vi "UHR-Fleezers Control (host) - 12.0.vi"() -> ()   [LabVIEW 2012] (continued)
      event "Reset Trap Pos. FB": Value Change {
        n2500 = event-data() -> ()  [unwired: 7 out]
        n2501 = xnode "Read/Write Control"("FPGA VI Reference In"=w4144, "error in"=w4143, "Trap Pos. FB Reset"="Reset Trap Pos. FB") -> ()  [unwired: 2 out]
      }
      event "Rem fb disp offset": Value Change {
        n2502 = event-data() -> ()  [unwired: 7 out]
        n2503 = local write "Rem fb disp offset"(FALSE ("Rem fb disp offset")) -> ()
        n2504 = local read "Mean T1 Position (nm)"() -> (w4146:dbl)
        n2505 = local read "FB Trap Pos Offset"() -> (w4147:dbl)
        n2506 = Subtract(x=w4147, y=w4146) -> (x-y=w4145:dbl)
        n2507 = local write "FB Trap Pos Offset"(w4145) -> ()
      }
      event "Threshold (nm)": Value Change {
        n2508 = event-data() -> ()  [unwired: 7 out]
        n2509 = flat-sequence {
          tunnel: w4151 -> [w4159]
          tunnel: w4150 -> [w4158]
          tunnel: [w4152] -> w4149
          tunnel: w4149 -> [w4165]
          frame #0 {
            n2510 = xnode "Read/Write Control"("FPGA VI Reference In"=w4159, "error in"=w4158) -> ("FPGA VI Reference Out"=w4155:T19, "error out"=w4154:errorcluster, "FPGA TTrig Thresh"=w4156:i64)
            n2511 = local read "Threshold stored (nm)"() -> (w4164:dbl)
            n2512 = local read "Threshold (nm)"() -> (w4152:dbl)
            n2513 = local read "AOM X Cal (nm/MHz)"() -> (w4162:dbl)
            n2514 = Subtract(x=w4152, y=w4164) -> (x-y=w4163:dbl)
            n2515 = Divide(x=w4163, y=w4162) -> (x/y=w4160:dbl)
            n2516 = call "IR AOM freq to word.vi"("Frequency In (MHz)"=w4160) -> ("Frequency Word Out (double)"=w4161:dbl)
            n2517 = To Quad Integer(1:w4161) -> (0:w4157:i64)
            n2518 = Add(x=w4156, y=w4157) -> (x+y=w4153:i64)
            n2519 = xnode "Read/Write Control"("FPGA VI Reference In"=w4155, "error in"=w4154, "FPGA TTrig Thresh"=w4153) -> ()  [unwired: 2 out]
          }
          frame #1 {
            "Threshold stored (nm)" <- w4165
          }
        }
      }
      event "FB Trig Integrate": Value Change {
        n2520 = event-data() -> ()  [unwired: 7 out]
        n2521 = local read "FB Trig Integrate"() -> (w4167:u32)
        n2522 = xnode "Read/Write Control"("FPGA VI Reference In"=w4169, "error in"=w4168, "FB Trig Integrate"=w4167) -> ("error out"=w4166:errorcluster)  [unwired: 1 out]
      }
      event "11": Value Change {
        n2523 = event-data() -> ()  [unwired: 7 out]
        n2524 = local read "11"() -> (w4170:bool)
        n2525 = case shown="True" w4170 {
          frame False {
          }
          frame True {
            n2526 = local read "Messages"() -> (w4172:string)
            n2527 = call "Update messages.vi"("Message to add"="You kicked it up to 11!", "Old message string"=w4172) -> ("New message string"=w4173:string)
            n2528 = call <vilib>:"Beep.vi"() -> ()  [unwired: 12 in]
            n2529 = local write "Messages"(w4173) -> ()
          }
        }
      }
      event "Trap Pos. FB ON": Value Change {
        n2530 = event-data() -> ()  [unwired: 7 out]
        n2531 = xnode "Read/Write Control"("FPGA VI Reference In"=w4176, "error in"=w4175, "Force feedback"="Trap Pos. FB ON") -> ()  [unwired: 2 out]
      }
      event "Remove Action Offset": Value Change {
        n2532 = event-data() -> ()  [unwired: 7 out]
        n2533 = local write "Remove Action Offset"(FALSE ("Remove Action Offset")) -> ()
        n2534 = local read "Trap Pos. FB Mult Factor"() -> (w4181:i64)
        n2535 = local read "Trap Pos FB Action"() -> (w4179:i64)
        n2536 = local read "Trap Pos. FB Offset Factor"() -> (w4177:i64)
        n2537 = Multiply(x=w4181, y=w4179) -> (x*y=w4180:i64)
        n2538 = Add(x=w4180, y=w4177) -> (x+y=w4178:i64)
        n2539 = local write "Trap Pos. FB Offset Factor"(w4178) -> ()
        n2540 = xnode "Read/Write Control"("FPGA VI Reference In"=w4184, "error in"=w4183, "Trap Pos. FB Offset Factor"=w4178) -> ()  [unwired: 2 out]
      }
      event "Remove Unwinding Offset": Value Change {
        n2541 = event-data() -> ()  [unwired: 7 out]
        n2542 = local write "Remove Unwinding Offset"(FALSE ("Remove Action Offset")) -> ()
        n2543 = local read "Trap Pos. FB Mult Factor"() -> (w4196:i64)
        n2544 = local read "Trap Pos FB Action"() -> (w4194:i64)
        n2545 = local read "Trap Pos. FB Offset Factor"() -> (w4193:i64)
        n2546 = Multiply(x=w4196, y=w4194) -> (x*y=w4195:i64)
        n2547 = local read "Trap Pos. FB Mult Factor"() -> (w4192:i64)
        n2548 = Add(x=w4195, y=w4193) -> (x+y=w4186:i64)
        n2549 = Multiply(x=32768, y="factor") -> (x*y=w4189:dbl)
        n2550 = Multiply(x=w4189, y=w4192) -> (x*y=w4191:dbl)
        n2551 = Subtract(x=w4186, y=w4191) -> (x-y=w4190:dbl)
        n2552 = To Quad Integer(1:w4190) -> (0:w4185:i64)
        n2553 = xnode "Read/Write Control"("FPGA VI Reference In"=w4199, "error in"=w4198, "Trap Pos. FB Offset Factor"=w4185) -> ()  [unwired: 2 out]
        n2554 = local write "Trap Pos. FB Offset Factor"(w4185) -> ()
      }
      event "Trap Pos. FB Range", "Trap Pos. FB Gains", "Trap Pos. FB Mult Factor", "Trap Pos. FB Offset Factor", "Trap Pos FB Negate Action", "Trap Pos FB Monitor\nT1 or T2", "Differential FB?", "Negate Diff?": Value Change {
        n2555 = event-data() -> ()  [unwired: 7 out]
        n2556 = local read "Negate Diff?"() -> (w4200:bool)
        n2557 = xnode "Read/Write Control"("FPGA VI Reference In"=w4210, "error in"=w4209, "Trap Pos. FB Range"="Trap Pos. FB Range", "Trap Pos. FB Gains"="Trap Pos. FB Gains", "Trap Pos. FB Mult Factor"="Trap Pos. FB Mult Factor", "Trap Pos. FB Offset Factor"="Trap Pos. FB Offset Factor", "Trap Pos FB Negate Action"="Trap Pos FB Negate Action", "Trap Pos FB Monitor T1 or T2"="Trap Pos FB Monitor\nT1 or T2", "AI1 X Scale"="Trap Pos. AI1 X Pre-scale", "Negate Diff?"=w4200, "Diff FB Measurement?"="Differential FB?") -> ()  [unwired: 2 out]
      }
      event "Trap Pos FB SP", "Trap Pos FB SP 2", "Use SP 2": Value Change {
        n2558 = event-data() -> ()  [unwired: 7 out]
        n2559 = Select(t="Trap Pos FB SP 2", s="Use SP 2", f="Trap Pos FB SP") -> (s? t:f=w4211:fxp<+/-,16,1>)
        n2560 = xnode "Read/Write Control"("FPGA VI Reference In"=w4216, "error in"=w4215, "Trap Pos. FB SP"=w4211) -> ()  [unwired: 2 out]
      }
      event "Offset SP2 from SP1": Value Change {
        n2561 = event-data() -> ()  [unwired: 7 out]
        n2562 = local read "Trap Pos FB SP"() -> (w4219:fxp<+/-,16,1>)
        n2563 = Add(x=w4219, y="SP2 Offset") -> (x+y=w4217:fxp<+/-,16,1>)
        n2564 = property on="Trap Pos FB SP 2" class="DigNum (strict)"("Val(Sgnl)"=w4217) -> ()  [unwired: 2 in, 2 out]
        n2565 = local write "Offset SP2 from SP1"(FALSE ("Offset SP2 from SP1")) -> ()
      }
      event "Set Reading to\nSetpoint": Value Change {
        # "This is the actual PID input signal"
        n2566 = event-data() -> ()  [unwired: 7 out]
        n2567 = local write "Set Reading to\nSetpoint"(FALSE ("Set SP to Reading")) -> ()
        n2568 = xnode "Read/Write Control"("FPGA VI Reference In"=w4225, "error in"=w4224) -> ("FPGA VI Reference Out"=w4223:T19, "error out"=w4222:errorcluster, "Trap Pos FB Int-Norm Signal"=w4221:fxp<+/-,16,1>)
        n2569 = local read "Differential FB?"() -> (w4226:bool)
        n2570 = case shown="False" w4226 {
          tunnel: [w4231 w4238] -> w4228
          tunnel: w4221 -> [w4229 w4238]
          frame False {
            n2571 = local read "Trap Pos FB Monitor\nT1 or T2"() -> (w4234:bool)
            n2572 = local read "Trap X AI1 (DMA)"() -> (w4237:T13)
            n2573 = Unbundle By Name(w4237) -> ("Set 1"=w4236:fxp<+/-,16,1>, "Set 2"=w4235:fxp<+/-,16,1>)
            n2574 = Select(t=w4236, s=w4234, f=w4235) -> (s? t:f=w4233:fxp<+/-,16,1>)
            n2575 = Not(x="Set SP Using...") -> (.not. x?=w4230:bool)
            n2576 = Select(t=w4229, s=w4230, f=w4233) -> (s? t:f=w4231:fxp<+/-,16,1>)
          }
          frame True {
          }
        }
        n2577 = xnode "Read/Write Control"("FPGA VI Reference In"=w4223, "error in"=w4222, "Trap Pos. FB SP"=w4228) -> ()  [unwired: 2 out]
        n2578 = local write "Trap Pos FB SP"(w4228) -> ()
      }
      event "Trap Pos. FB Out Scale 2^n": Value Change {
        n2579 = event-data() -> ()  [unwired: 7 out]
        n2580 = Scale By Power Of 2(n="Trap Pos. FB Out Scale 2^n", x=ext 1.0) -> (x*2^n=w4239:ext)
        n2581 = property on="Trap Pos. FB Mult Factor" class="DigNum (strict)"("Val(Sgnl)"=w4239) -> ()  [unwired: 2 in, 2 out]
      }
      event "Trap Pos FB Int Count": Value Change {
        n2582 = event-data() -> ()  [unwired: 7 out]
        n2583 = xnode "Read/Write Control"("FPGA VI Reference In"=w4244, "error in"=w4243, "Trap Pos FB Int Count"="Trap Pos FB Int Count") -> ()  [unwired: 2 out]
      }
      event "Trap pos": Value Change {
        n2584 = event-data() -> ()  [unwired: 7 out]
        n2585 = case shown="True" "Trap pos" {
          frame False {
            n2586 = property on="Trap Delta Graph" class="WFGraph (strict)"("Visible"=TRUE) -> ()  [unwired: 2 in, 2 out]
            n2587 = property on="Saved trap pos" class="WFGraph (strict)"("Visible"=FALSE) -> ()  [unwired: 2 in, 2 out]
          }
          frame True {
            n2588 = property on="Saved trap pos" class="WFGraph (strict)"("Visible"=TRUE) -> ()  [unwired: 2 in, 2 out]
            n2589 = property on="Trap Delta Graph" class="WFGraph (strict)"("Visible"=FALSE) -> ()  [unwired: 2 in, 2 out]
          }
        }
      }
    }
    "error out 2" <- w3149
    n2590 = node-c288() -> ()  [unwired: 2 out]
  }
  n2591 = timed-loop "Oscillate Trap/AOM (fishing, debugging)" {
    tunnel: w6 -> [w4251]
    tunnel: [w4250] -> w100
    timing: w95 -> [_]
    timing-out: [_] -> w94
    stop <- w4250 stop-if-true
    n2592 = node-c288() -> ()  [unwired: 2 out]
    n2593 = event shown="[0] \"Oscillate Set 1\", \"Fish for Tether\": Value Change" {
      selector: _ -> [_ _ _]
      dyn-events: _ -> [_ _ _]
      timeout: _ -> [_ _ _]
      tunnel: w4251 -> [w4258 _ _]
      tunnel: [FALSE ("Stop All") _ w4847] -> w4250
      event "Oscillate Set 1", "Fish for Tether": Value Change {
        n2594 = event-data() -> ()  [unwired: 6 out]
        n2595 = local read "Oscillate Set 1"() -> (w4257:bool)
        n2596 = Or(x=w4257, y="Fish for Tether") -> (x .or. y?=w4255:bool)
        n2597 = case shown="True" w4255 {
          tunnel: w4258 -> [_ w4261]
          tunnel: "Fish for Tether" -> [_ w4260]
          frame False {
          }
          frame True {
            n2598 = case shown="True" w4260 {
              selector: w4260 -> [w4264 w4270]
              tunnel: [w4264 w4270] -> w4259
              frame False {
              }
              frame True {
                n2599 = local write "Scan axis 2"(TRUE) -> ()
                n2600 = local write "Tether"(FALSE ("Tether")) -> ()
                n2601 = local read "Flow ON during cal?"() -> (w4265:bool)
                n2602 = property on="Trap Delta (MHz)" class="DigNum (strict)"("Val(Sgnl)"="Furthest Delta (MHz)") -> ()  [unwired: 2 in, 2 out]
                n2603 = Or(x="Flow ON during \nfishing?", y=w4265) -> (x .or. y?=w4266:bool)
                n2604 = Wait (ms)(milliseconds to wait=u32 500) -> ()  [unwired: 1 out]
                n2605 = property on="Sample Channel\nFlow" class="Bool (strict)"("Val(Sgnl)"=w4266) -> ()  [unwired: 2 in, 2 out]
              }
            }
            n2606 = node-c288() -> (w4263:T21)  [unwired: 4 out]
            n2607 = timed-loop "Oscillate AOD" {
              timing: w4263 -> [_]
              timing-out: [_] -> w4262
              tunnel: w4261 -> [w4280]
              tunnel: w4259 -> [w4273]
              i -> [w4282]
              stop <- w4279 stop-if-true
              n2608 = node-c288() -> (w4281:i64)  [unwired: 1 out]
              n2609 = flat-sequence {
                tunnel: w4282 -> [w4309]
                tunnel: w4281 -> [w4308]
                tunnel: w4280 -> [w4287]
                tunnel: w4273 -> [w4290]
                tunnel: [w4290] -> w4278
                tunnel: [w4289] -> w4277
                tunnel: [w4286] -> w4276
                tunnel: [w4283] -> w4274
                tunnel: w4278 -> [w4345]
                tunnel: w4277 -> [w4343]
                tunnel: w4276 -> [w4342]
                tunnel: [w4341] -> w4275
                tunnel: w4274 -> [w4340]
                tunnel: [w4417] -> w4279
                tunnel: w4275 -> [w4416]
                frame #0 {
                  n2610 = Divide(x=w4308, y=i64 1000) -> (x/y=w4303:dbl)
                  n2611 = Multiply(x=w4303, y=w4309) -> (x*y=w4305:dbl)
                  n2612 = local read "BD 1 Frequency 2 (MHz)"() -> (w4288:dbl)
                  n2613 = Multiply(x="Osc. freq. (Hz)", y=6.283185307179586) -> (x*y=w4306:dbl)
                  n2614 = Multiply(x=w4306, y=w4305) -> (x*y=w4285:dbl)
                  n2615 = local read "BD 1 Frequency 1 (MHz)"() -> (w4293:dbl)
                  n2616 = local read "BD 2 Frequency 1 (MHz)"() -> (w4292:dbl)
                  n2617 = case shown="True" w4290 {
                    tunnel: w4285 -> [w4315 w4320]
                    tunnel: w4293 -> [_ w4331]
                    tunnel: w4288 -> [_ w4332]
                    tunnel: [w4312 w4326] -> w4291
                    tunnel: [FALSE w4323] -> w4286
                    tunnel: [0.0 w4316] -> w4283
                    frame False {
                      n2618 = Sine(x=w4315) -> (sin(x)=w4313:dbl)
                      n2619 = Multiply(x=w4313, y="Osc. amp. (MHz)") -> (x*y=w4312:dbl)
                    }
                    frame True {
                      n2620 = Cosine(x=w4320) -> (cos(x)=w4335:dbl)
                      n2621 = Subtract(x=w4332, y=w4331) -> (x-y=w4330:dbl)
                      n2622 = Decrement(x=w4335) -> (x-1=w4334:dbl)
                      n2623 = Subtract(x=w4330, y="Closest Delta (MHz)") -> (x-y=w4327:dbl)
                      n2624 = Divide(x=w4334, y=-2.0) -> (x/y=w4328:dbl)
                      n2625 = Multiply(x=w4328, y=w4327) -> (x*y=w4326:dbl)
                      n2626 = local read "Vec Mean of T1 T2"() -> (w4322:dbl[])
                      n2627 = Greater?(x=w4322, y="Stop F (pN)") -> (0:w4324:bool[])
                      n2628 = Or Array Elements(Boolean array=w4324) -> (logical OR=w4323:bool)
                      n2629 = Divide(x=w4320, y=6.283185307179586) -> (x/y=w4319:dbl)
                      n2630 = Round Toward +Infinity(x=w4319) -> (ceil(x): smallest int >= x=w4316:dbl)
                      "Attempts" <- w4316
                      n2631 = Greater?(x=w4316, y="Attempt Limit") -> (0:w4318:bool)
                      n2632 = case shown="True" w4318 {
                        frame False {
                        }
                        frame True {
                          n2633 = local write "Fish for Tether"(FALSE ("Fish for Tether")) -> ()
                          n2634 = call <vilib>:"Beep.vi"() -> ()  [unwired: 3 in, 9 out]
                          n2635 = local read "Messages"() -> (w4337:string)
                          n2636 = call "Update messages.vi"("Message to add"="Tether fishing timeout." ("Messages"), "Old message string"=w4337) -> ("New message string"=→"Messages":string)
                        }
                      }
                    }
                  }
                  n2637 = Select(t=w4293, s="Scan axis 2", f=w4292) -> (s? t:f=w4296:dbl)
                  n2638 = Add(x=w4291, y=w4296) -> (x+y=w4289:dbl)
                  n2639 = Select(t=w4289, s="Scan axis 2", f=w4293) -> (s? t:f=w4299:dbl)
                  n2640 = Select(t=w4292, s="Scan axis 2", f=w4289) -> (s? t:f=w4298:dbl)
                  n2641 = local read "Y RF Frequency Limits (MHz)"() -> (w4294:T16)
                  n2642 = local read "X RF Frequency Limits (MHz)"() -> (w4295:T16)
                  n2643 = local read "BD 1 Frequency 3 (MHz)"() -> (w4302:dbl)
                  n2644 = local read "BD 2 Frequency 2 (MHz)"() -> (w4301:dbl)
                  n2645 = local read "BD 2 Frequency 3 (MHz)"() -> (w4300:dbl)
                  n2646 = call "set RF board frequency - interlace.vi"("Board 2 Frequency Limits"=w4294, "Board 1 Frequency Limits"=w4295, "FPGA VI Reference In"=w4287, "Board 2 Frequency 3 (MHz)"=w4300, "Board 1 Frequency 3 (MHz)"=w4302, "Board 2 Frequency 2 (MHz)"=w4301, "Board 2 Frequency 1 (MHz)"=w4298, "Board 1 Frequency 2 (MHz)"=w4288, "Board 1 Frequency 1  (MHz)"=w4299) -> ()  [unwired: 1 in, 2 out]
                }
                frame #1 {
                  n2647 = And(x=w4345, y=w4342) -> (x .and. y?=w4344:bool)
                  n2648 = case "Only if were fishing and now formed tether" shown="False" w4344 {
                    tunnel: w4343 -> [w4347 w4362]
                    tunnel: [w4346 w4361] -> w4341
                    tunnel: w4340 -> [_ w4357]
                    frame False {
                      n2649 = local read "Fish for Tether"() -> (w4346:bool)
                      n2650 = case shown="False" w4346 {
                        tunnel: w4347 -> [w4348 _]
                        frame False {
                          n2651 = property on="BD 1 Frequency 1 (MHz)" class="DigNum (strict)"("Val(Sgnl)"=w4348) -> ()  [unwired: 2 in, 2 out]
                        }
                        frame True {
                        }
                      }
                    }
                    frame True {
                      w4361 = FALSE ("Fish for Tether")
                      n2652 = call <vilib>:"Beep.vi"() -> ()  [unwired: 3 in, 9 out]
                      n2653 = Number To Decimal String(number=w4357, width (-)=i16 1) -> (decimal integer string=w4355:string)
                      n2654 = Concatenate Strings("Formed tether in ", w4355, " attempt(s)." ("string")) -> (w4352:string)
                      n2655 = local read "Messages"() -> (w4359:string)
                      n2656 = local write "Fish for Tether"(w4361) -> ()
                      n2657 = call "Update messages.vi"("Message to add"=w4352, "Old message string"=w4359) -> ("New message string"=w4358:string)
                      n2658 = local write "Messages"(w4358) -> ()
                      n2659 = Get Date/Time In Seconds() -> (seconds since 1Jan1904=→"Time tether formed":timestamp)
                      n2660 = local read "Flow ON during cal?"() -> (w4349:bool)
                      n2661 = property on="Sample Channel\nFlow" class="Bool (strict)"("Val(Sgnl)"=w4349) -> (error out=w4350:errorcluster)  [unwired: 2 in, 1 out]
                      n2662 = case shown="\"2\", \"3\", \"4\", \"5\", \"6\"" "Then..." {
                        selector: "Then..." -> [_ w4365]
                        tunnel: w4362 -> [w4364 _]
                        tunnel: w4350 -> [_ _]
                        frame "1", Default {
                          n2663 = property on="BD 1 Frequency 1 (MHz)" class="DigNum (strict)"("Val(Sgnl)"=w4364) -> ()  [unwired: 2 in, 2 out]
                        }
                        frame "2", "3", "4", "5", "6" {
                          n2664 = flat-sequence {
                            tunnel: w4365 -> [w4367]
                            frame #0 {
                              n2665 = property on="Trap Delta (MHz)" class="DigNum (strict)"("Val(Sgnl)"="Move to Delta 1 (MHz)") -> ()  [unwired: 2 in, 2 out]
                            }
                            frame #1 {
                              n2666 = case shown="\"5\", \"6\"" w4367 {
                                selector: w4367 -> [w4370 w4380 _]
                                frame "3", "4" {
                                n2667 = flat-sequence {
                                tunnel: w4370 -> [w4371]
                                tunnel: [w4371] -> w4368
                                tunnel: [w4373] -> w4369
                                tunnel: w4368 -> [w4373]
                                tunnel: w4369 -> [w4377]
                                frame #0 {
                                n2668 = property on="Green Laser ON/Interlacing" class="Bool (strict)"("Val(Sgnl)"=TRUE ("Value (Signaling)")) -> ()  [unwired: 2 in, 2 out]
                                }
                                frame #1 {
                                n2669 = Multiply(x="Wait Before Save (s)", y=u32 1000 ("x")) -> (x*y=w4375:u32)
                                n2670 = Wait (ms)(milliseconds to wait=w4375) -> ()  [unwired: 1 out]
                                }
                                frame #2 {
                                n2671 = property on="Start Saving" class="Bool (strict)"("Value"=TRUE ("Start Saving")) -> ()  [unwired: 2 in, 2 out]
                                n2672 = case shown="\"4\"" w4377 {
                                frame Default {
                                }
                                frame "4" {
                                n2673 = property on="Fl. Triggered..." class="Bool (strict)"("Val(Sgnl)"=TRUE ("Value (Signaling)")) -> ()  [unwired: 2 in, 2 out]
                                }
                                }
                                }
                                }
                                }
                                frame "5", "6" {
                                n2674 = stacked-sequence {
                                tunnel: w4380 -> [_ _ _ _ _ _ w4392]
                                frame #0 {
                                n2675 = Replace Array Subset(array=u32[] [0] ("Index Values"), new element="Raster Set Upon Tether", index=0) -> (w4381:u32[])
                                n2676 = property on="Saved AOD Raster Scan Parameter Sets" class="Arr (strict)"("Index Values"=w4381) -> ()  [unwired: 2 in, 2 out]
                                }
                                frame #1 {
                                n2677 = Wait (ms)(milliseconds to wait=u32 500) -> ()  [unwired: 1 out]
                                }
                                frame #2 {
                                n2678 = property on="Load parameters" class="Bool (strict)"("Val(Sgnl)"=TRUE ("Value (Signaling)")) -> ()  [unwired: 2 in, 2 out]
                                n2679 = case shown="True" "Green ON During Raster" {
                                frame False {
                                }
                                frame True {
                                n2680 = property on="Green Laser ON/Interlacing" class="Bool (strict)"("Val(Sgnl)"=TRUE ("Value (Signaling)")) -> ()  [unwired: 2 in, 2 out]
                                }
                                }
                                }
                                frame #3 {
                                n2681 = Wait (ms)(milliseconds to wait=u32 500) -> ()  [unwired: 1 out]
                                }
                                frame #4 {
                                n2682 = property on="Trap Raster Scan" class="Bool (strict)"("Val(Sgnl)"=TRUE ("Value (Signaling)")) -> ()  [unwired: 2 in, 2 out]
                                }
                                frame #5 {
                                n2683 = Wait (ms)(milliseconds to wait=u32 2000) -> ()  [unwired: 1 out]
                                }
                                frame #6 {
                                n2684 = flat-sequence {
                                tunnel: w4392 -> [w4399]
                                frame #0 {
                                n2685 = while {
                                stop <- w4395 stop-if-true
                                n2686 = local read "Raster Scanning..."() -> (w4394:bool)
                                n2687 = local read "Saving..."() -> (w4397:bool)
                                n2688 = Wait (ms)(milliseconds to wait=u32 100) -> ()  [unwired: 1 out]
                                n2689 = Not(x=w4397) -> (.not. x?=w4396:bool)
                                n2690 = Not(x=w4394) -> (.not. x?=w4393:bool)
                                n2691 = And(x=w4396, y=w4393) -> (x .and. y?=w4395:bool)
                                }
                                }
                                frame #1 {
                                n2692 = local read "Tether"() -> (w4400:bool)
                                n2693 = case shown="True" w4400 {
                                tunnel: w4399 -> [_ w4402]
                                frame False {
                                n2694 = property on="Fish for Tether" class="Bool (strict)"("Val(Sgnl)"="Fish again after \nraster break?") -> ()  [unwired: 2 in, 2 out]
                                }
                                frame True {
                                n2695 = stacked-sequence {
                                tunnel: w4402 -> [_ w4406 _ _]
                                frame #0 {
                                n2696 = property on="Trap Delta (MHz)" class="DigNum (strict)"("Val(Sgnl)"="Move to Delta 2 (MHz)") -> ()  [unwired: 2 in, 2 out]
                                n2697 = case shown="True" "Flow ON after\ntether testing?" {
                                frame False {
                                }
                                frame True {
                                n2698 = property on="Sample Channel\nFlow" class="Bool (strict)"("Val(Sgnl)"=TRUE ("Value (Signaling)")) -> ()  [unwired: 2 in, 2 out]
                                }
                                }
                                }
                                frame #1 {
                                n2699 = flat-sequence {
                                tunnel: w4406 -> [w4408]
                                frame #0 {
                                n2700 = Wait (ms)(milliseconds to wait=u32 500) -> ()  [unwired: 1 out]
                                }
                                frame #1 {
                                n2701 = case shown="\"6\"" w4408 {
                                frame Default {
                                }
                                frame "6" {
                                n2702 = property on="Green Laser ON/Interlacing" class="Bool (strict)"("Val(Sgnl)"=TRUE ("Green Laser ON/Interlacing")) -> ()  [unwired: 2 in, 2 out]
                                }
                                }
                                }
                                frame #2 {
                                n2703 = Wait (ms)(milliseconds to wait=u32 500) -> ()  [unwired: 1 out]
                                }
                                frame #3 {
                                n2704 = local write "Start Saving"("Save at end (5, 6)") -> ()
                                }
                                }
                                }
                                frame #2 {
                                n2705 = local read "Bead Sep. Int. Time (s)"() -> (w4414:dbl)
                                n2706 = Multiply(x=w4414, y=1000.0) -> (x*y=w4413:dbl)
                                n2707 = Wait (ms)(milliseconds to wait=w4413) -> ()  [unwired: 1 out]
                                }
                                frame #3 {
                                n2708 = property on="Remove Offset" class="Bool (strict)"("Val(Sgnl)"=TRUE ("Value (Signaling)")) -> ()  [unwired: 2 in, 2 out]
                                }
                                }
                                }
                                }
                                }
                                }
                                }
                                }
                                }
                                frame "2", Default {
                                }
                              }
                            }
                          }
                        }
                      }
                      "Tether" <- "Tether Alarm?"
                    }
                  }
                }
                frame #2 {
                  n2709 = local read "Oscillate Set 1"() -> (w4421:bool)
                  n2710 = local read "Stop All"() -> (w4419:bool)
                  n2711 = Or(x=w4421, y=w4416) -> (x .or. y?=w4418:bool)
                  n2712 = Not(x=w4418) -> (.not. x?=w4420:bool)
                  n2713 = Compound Arithmetic op=OR(w4419, w4420) -> (w4417:bool)
                }
              }
              n2714 = node-c288() -> ()  [unwired: 2 out]
            }
            n2715 = node-c288(w4262) -> ()  [unwired: 1 out]
          }
        }
      }
      event "Fl. Triggered...": Value Change {
        n2716 = event-data() -> ()  [unwired: 7 out]
        n2717 = case shown="True" "Fl. Triggered..." {
          frame False {
          }
          frame True {
            n2718 = node-c288() -> (w4432:T21)  [unwired: 4 out]
            n2719 = timed-loop {
              timing: w4432 -> [_]
              timing-out: [_] -> w4431
              tunnel: "Action" -> [w4440]
              shift-right: [w4437] -> _
              shift-left: u8 255 -> [w4439]
              shift-right: [w4434] -> _
              shift-left: 255 -> [w4436]
              stop <- w4433 stop-if-true
              # "Reset confocal spot"
              n2720 = node-c288() -> ()  [unwired: 2 out]
              n2721 = flat-sequence {
                tunnel: w4440 -> [w4460]
                tunnel: w4439 -> [w4459]
                tunnel: [w4458] -> w4438
                tunnel: w4436 -> [w4445]
                tunnel: [w4444] -> w4435
                tunnel: [w4839] -> w4433
                tunnel: w4438 -> [w4838]
                tunnel: [w4838] -> w4437
                tunnel: [w4837] -> w4434
                tunnel: w4435 -> [w4837]
                frame #0 {
                  n2722 = local read "Delta Fl. 2"() -> (w4457:dbl)
                  n2723 = local read "Delta Fl. 1"() -> (w4452:dbl)
                  n2724 = Multiply(x="Fl. Delta Thresh. (kHz)", y=1000.0) -> (x*y=w4447:dbl)
                  n2725 = Select(t=w4452, s="APD to Watch", f=w4457) -> (s? t:f=w4448:dbl)
                  n2726 = Greater?(x=w4448, y=w4447) -> (0:w4453:bool)
                  n2727 = Or(x="Force Yank", y=w4453) -> (x .or. y?=w4451:bool)
                  n2728 = And(x=w4451, y="Yank when?") -> (x .and. y?=w4449:bool)
                  n2729 = case shown="False" w4449 {
                    tunnel: w4460 -> [w4463 w4664]
                    tunnel: w4459 -> [w4465 w4660]
                    tunnel: [w4465 w4658] -> w4458
                    tunnel: w4448 -> [w4471 _]
                    tunnel: w4447 -> [w4470 _]
                    tunnel: "Force Yank" -> [w4468 _]
                    tunnel: w4445 -> [w4467 w4657]
                    tunnel: [w4466 w4657] -> w4444
                    frame False {
                      n2730 = Negate(x=w4470) -> (-x=w4462:dbl)
                      n2731 = local write "Fl. High"(TRUE ("Fl. High")) -> ()
                      n2732 = Less?(x=w4471, y=w4462) -> (x < y?=w4469:bool)
                      n2733 = Or(x=w4468, y=w4469) -> (x .or. y?=w4464:bool)
                      n2734 = case shown="True" w4464 {
                        tunnel: w4467 -> [w4472 w4482]
                        tunnel: [w4472 w4481] -> w4466
                        tunnel: w4463 -> [_ w4480]
                        frame False {
                        }
                        frame True {
                          n2735 = flat-sequence {
                            tunnel: w4482 -> [w4488]
                            tunnel: w4480 -> [w4485]
                            tunnel: [w4487] -> w4479
                            tunnel: [w4486] -> w4478
                            tunnel: [w4485] -> w4477
                            tunnel: w4476 -> [w4484]
                            tunnel: [w4484] -> w4475
                            tunnel: w4474 -> [w4483]
                            tunnel: [w4483] -> w4473
                            tunnel: [w4559] -> w4481
                            tunnel: w4479 -> [w4559]
                            tunnel: w4478 -> [w4558]
                            tunnel: w4477 -> [w4557]
                            tunnel: w4475 -> [w4556]
                            tunnel: w4473 -> [w4555]
                            frame #0 {
                              n2736 = call <vilib>:"Beep.vi"() -> ()  [unwired: 12 in]
                              n2737 = local write "Waiting"(FALSE ("Waiting")) -> ()
                              n2738 = Increment(x=w4488) -> (x+1=w4487:i32)
                              n2739 = case shown="\"Yank\"" w4485 {
                                tunnel: w4487 -> [_ w4493 _]
                                frame "Alarm", Default {
                                }
                                frame "Yank" {
                                n2740 = flat-sequence {
                                tunnel: w4493 -> [w4496]
                                tunnel: [w4495] -> w4492
                                tunnel: [w4494] -> w4491
                                tunnel: w4492 -> [w4506]
                                tunnel: w4491 -> [w4507]
                                frame #0 {
                                n2741 = local read "Yank Delay (s)"() -> (w4499:dbl)
                                n2742 = local read "N Array El"() -> (w4494:u8)
                                n2743 = Quotient & Remainder(x=w4496, y=w4494) -> (x-y*floor(x/y)=w4495:i32)  [unwired: 1 out]
                                n2744 = Multiply(x=w4499, y=1000.0) -> (x*y=w4497:dbl)
                                n2745 = Wait (ms)(milliseconds to wait=w4497) -> ()  [unwired: 1 out]
                                }
                                frame #1 {
                                n2746 = local read "Yank to which?"() -> (w4501:bool)
                                n2747 = local read "Random Choice"() -> (w4511:bool)
                                n2748 = local read "Yank to Trap Delta (MHz)"() -> (w4504:dbl[])
                                n2749 = local read "Yank to SP"() -> (w4505:dbl[])
                                n2750 = Random Number (0-1)() -> (number: 0 to 1=w4510:dbl)
                                n2751 = Multiply(x=w4507, y=w4510) -> (x*y=w4509:dbl)
                                n2752 = Round Toward -Infinity(1:w4509) -> (0:w4508:dbl)
                                n2753 = Select(t=w4508, s=w4511, f=w4506) -> (s? t:f=w4502:dbl)
                                n2754 = Select(t=w4504, s=w4501, f=w4505) -> (s? t:f=w4503:dbl[])
                                n2755 = Index Array(array=w4503, index=w4502) -> (element=w4500:dbl)
                                n2756 = case shown="True" w4501 {
                                tunnel: w4500 -> [w4512 w4539]
                                frame False {
                                n2757 = flat-sequence {
                                tunnel: w4512 -> [w4513]
                                frame #0 {
                                n2758 = property on="Trap Pos FB SP" class="DigNum (strict)"("Val(Sgnl)"=w4513) -> ()  [unwired: 2 in, 2 out]
                                }
                                frame #1 {
                                n2759 = Wait (ms)(milliseconds to wait=u32 700) -> ()  [unwired: 1 out]
                                }
                                frame #2 {
                                n2760 = local read "Action (%)"() -> (w4518:dbl)
                                n2761 = Absolute Value(x=w4518) -> (abs(x)=w4517:dbl)
                                n2762 = Greater?(x=w4517, y=70.0) -> (0:w4515:bool)
                                n2763 = property on="Remove Action Offset" class="Bool (strict)"("Val(Sgnl)"=w4515) -> ()  [unwired: 2 in, 2 out]
                                }
                                frame #3 {
                                n2764 = for {
                                N: 4 -> [_]
                                n2765 = flat-sequence {
                                frame #0 {
                                n2766 = Wait (ms)(milliseconds to wait=u32 500) -> ()  [unwired: 1 out]
                                }
                                frame #1 {
                                n2767 = local read "Action (%)"() -> (w4524:dbl)
                                n2768 = Absolute Value(x=w4524) -> (abs(x)=w4523:dbl)
                                n2769 = Greater?(x=w4523, y=70.0) -> (0:w4521:bool)
                                n2770 = property on="Remove Action Offset" class="Bool (strict)"("Val(Sgnl)"=w4521) -> ()  [unwired: 2 in, 2 out]
                                }
                                }
                                }
                                }
                                frame #4 {
                                n2771 = Wait (ms)(milliseconds to wait=u32 500) -> ()  [unwired: 1 out]
                                }
                                frame #5 {
                                n2772 = local read "Mean"() -> (w4532:dbl)
                                n2773 = Greater?(x=w4532, y=11.0) -> (0:w4526:bool)
                                n2774 = Not(x=w4526) -> (.not. x?=w4527:bool)
                                n2775 = And(x=w4527, y="Shift confocal") -> (x .and. y?=w4529:bool)
                                n2776 = And(x=w4526, y="Shift confocal") -> (x .and. y?=w4530:bool)
                                n2777 = case shown="True" w4530 {
                                frame False {
                                }
                                frame True {
                                n2778 = local read "Confocal Y 2 (V)"() -> (w4536:dbl)
                                n2779 = local read "Confocal X 2 (V)"() -> (w4535:dbl)
                                n2780 = property on="AO1" class="Slide (strict)"("Val(Sgnl)"=w4536) -> ()  [unwired: 2 in, 2 out]
                                n2781 = property on="AO2" class="Slide (strict)"("Val(Sgnl)"=w4535) -> ()  [unwired: 2 in, 2 out]
                                }
                                }
                                n2782 = case shown="True" w4529 {
                                frame False {
                                }
                                frame True {
                                n2783 = local read "Confocal Y 1 (V)"() -> (w4534:dbl)
                                n2784 = local read "Confocal X 1 (V)"() -> (w4533:dbl)
                                n2785 = property on="AO1" class="Slide (strict)"("Val(Sgnl)"=w4534) -> ()  [unwired: 2 in, 2 out]
                                n2786 = property on="AO2" class="Slide (strict)"("Val(Sgnl)"=w4533) -> ()  [unwired: 2 in, 2 out]
                                }
                                }
                                }
                                frame #6 {
                                n2787 = Wait (ms)(milliseconds to wait=u32 1500) -> ()  [unwired: 1 out]
                                }
                                frame #7 {
                                n2788 = property on="Rem fb disp offset" class="Bool (strict)"("Val(Sgnl)"=TRUE ("Value (Signaling)")) -> ()  [unwired: 2 in, 2 out]
                                }
                                }
                                }
                                frame True {
                                n2789 = flat-sequence {
                                tunnel: w4539 -> [w4540]
                                frame #0 {
                                n2790 = property on="Trap Delta (MHz)" class="DigNum (strict)"("Val(Sgnl)"=w4540) -> ()  [unwired: 2 in, 2 out]
                                }
                                frame #1 {
                                n2791 = Wait (ms)(milliseconds to wait=u32 500) -> ()  [unwired: 1 out]
                                }
                                frame #2 {
                                n2792 = local read "Shift confocal"() -> (w4546:bool)
                                n2793 = local read "Mean"() -> (w4548:dbl)
                                n2794 = Greater?(x=w4548, y=11.0) -> (0:w4545:bool)
                                n2795 = Not(x=w4545) -> (.not. x?=w4544:bool)
                                n2796 = And(x=w4544, y=w4546) -> (x .and. y?=w4542:bool)
                                n2797 = And(x=w4545, y=w4546) -> (x .and. y?=w4543:bool)
                                n2798 = case shown="True" w4543 {
                                frame False {
                                }
                                frame True {
                                n2799 = local read "Confocal Y 2 (V)"() -> (w4552:dbl)
                                n2800 = local read "Confocal X 2 (V)"() -> (w4551:dbl)
                                n2801 = property on="AO2" class="Slide (strict)"("Val(Sgnl)"=w4551) -> ()  [unwired: 2 in, 2 out]
                                n2802 = property on="AO1" class="Slide (strict)"("Val(Sgnl)"=w4552) -> ()  [unwired: 2 in, 2 out]
                                }
                                }
                                n2803 = case shown="True" w4542 {
                                frame False {
                                }
                                frame True {
                                n2804 = local read "Confocal X 1 (V)"() -> (w4549:dbl)
                                n2805 = local read "Confocal Y 1 (V)"() -> (w4550:dbl)
                                n2806 = property on="AO2" class="Slide (strict)"("Val(Sgnl)"=w4549) -> ()  [unwired: 2 in, 2 out]
                                n2807 = property on="AO1" class="Slide (strict)"("Val(Sgnl)"=w4550) -> ()  [unwired: 2 in, 2 out]
                                }
                                }
                                }
                                }
                                }
                                }
                                }
                                }
                                }
                                frame "Image" {
                                n2808 = property on="Confocal Image" class="Bool (strict)"("Val(Sgnl)"=TRUE ("Value (Signaling)")) -> ()  [unwired: 2 in, 2 out]
                                }
                              }
                              n2809 = local write "Fl. High"(FALSE ("Fl. High")) -> ()
                              n2810 = local read "Time (s)"() -> (w4486:dbl)
                            }
                            frame #1 {
                              n2811 = case shown="True" "Auto F Reset" {
                                tunnel: w4558 -> [_ w4563]
                                tunnel: w4557 -> [_ w4562]
                                tunnel: w4556 -> [_ w4561]
                                tunnel: w4555 -> [_ w4560]
                                frame False {
                                }
                                frame True {
                                n2812 = node-c288() -> (w4565:T21)  [unwired: 4 in]
                                n2813 = timed-loop {
                                timing: w4565 -> [_]
                                timing-out: [_] -> w4564
                                tunnel: w4563 -> [w4570]
                                tunnel: w4562 -> [w4569]
                                tunnel: w4561 -> [w4568]
                                tunnel: w4560 -> [w4567]
                                stop <- w4566 stop-if-true
                                n2814 = node-c288() -> ()  [unwired: 1 in, 1 out]
                                n2815 = local read "Fl. Delta Thresh. (kHz)"() -> (w4579:dbl)
                                n2816 = local read "APD to Watch"() -> (w4580:bool)
                                n2817 = local read "Delta Fl. 1"() -> (w4581:dbl)
                                n2818 = local read "Delta Fl. 2"() -> (w4582:dbl)
                                n2819 = local read "Fl. Triggered..."() -> (w4573:bool)
                                n2820 = local read "Stop All"() -> (w4574:bool)
                                n2821 = local read "Reset Force"() -> (w4572:bool)
                                n2822 = Multiply(x=w4579, y=1000.0) -> (x*y=w4577:dbl)
                                n2823 = Not(x=w4573) -> (.not. x?=w4571:bool)
                                n2824 = Select(t=w4581, s=w4580, f=w4582) -> (s? t:f=w4576:dbl)
                                n2825 = Greater?(x=w4576, y=w4577) -> (0:w4575:bool)
                                n2826 = Compound Arithmetic op=OR(w4575, w4574, w4571, w4572) -> (w4566:bool)
                                n2827 = case shown="True" w4566 {
                                tunnel: w4570 -> [_ w4586]
                                tunnel: w4569 -> [_ w4590]
                                tunnel: w4568 -> [_ w4589]
                                tunnel: w4567 -> [_ w4588]
                                frame False {
                                }
                                frame True {
                                n2828 = case shown="\"Yank\"" w4590 {
                                tunnel: w4589 -> [_ w4600]
                                tunnel: w4588 -> [_ w4598]
                                frame "Image", Default {
                                }
                                frame "Yank" {
                                n2829 = flat-sequence {
                                tunnel: [w4603] -> w4601
                                tunnel: w4600 -> [w4603]
                                tunnel: [w4602] -> w4599
                                tunnel: w4598 -> [w4602]
                                tunnel: w4601 -> [w4609]
                                tunnel: w4599 -> [w4607]
                                frame #0 {
                                n2830 = local read "Yank Delay (s)"() -> (w4606:dbl)
                                n2831 = Multiply(x=w4606, y=1000.0) -> (x*y=w4604:dbl)
                                n2832 = Wait (ms)(milliseconds to wait=w4604) -> ()  [unwired: 1 out]
                                }
                                frame #1 {
                                n2833 = local read "Yank to which?"() -> (w4608:bool)
                                n2834 = case shown="False" w4608 {
                                tunnel: w4609 -> [_ w4637]
                                tunnel: w4607 -> [w4610 _]
                                frame False {
                                n2835 = flat-sequence {
                                tunnel: w4610 -> [w4611]
                                frame #0 {
                                n2836 = property on="Trap Pos FB SP" class="DigNum (strict)"("Val(Sgnl)"=w4611) -> ()  [unwired: 2 in, 2 out]
                                }
                                frame #1 {
                                n2837 = Wait (ms)(milliseconds to wait=u32 700) -> ()  [unwired: 1 out]
                                }
                                frame #2 {
                                n2838 = local read "Action (%)"() -> (w4616:dbl)
                                n2839 = Absolute Value(x=w4616) -> (abs(x)=w4615:dbl)
                                n2840 = Greater?(x=w4615, y=70.0) -> (0:w4613:bool)
                                n2841 = property on="Remove Action Offset" class="Bool (strict)"("Val(Sgnl)"=w4613) -> ()  [unwired: 2 in, 2 out]
                                }
                                frame #3 {
                                n2842 = for {
                                N: 4 -> [_]
                                n2843 = flat-sequence {
                                frame #0 {
                                n2844 = Wait (ms)(milliseconds to wait=u32 500) -> ()  [unwired: 1 out]
                                }
                                frame #1 {
                                n2845 = local read "Action (%)"() -> (w4622:dbl)
                                n2846 = Absolute Value(x=w4622) -> (abs(x)=w4621:dbl)
                                n2847 = Greater?(x=w4621, y=70.0) -> (0:w4619:bool)
                                n2848 = property on="Remove Action Offset" class="Bool (strict)"("Val(Sgnl)"=w4619) -> ()  [unwired: 2 in, 2 out]
                                }
                                }
                                }
                                }
                                frame #4 {
                                n2849 = Wait (ms)(milliseconds to wait=u32 500) -> ()  [unwired: 1 out]
                                }
                                frame #5 {
                                n2850 = local read "Shift confocal"() -> (w4627:bool)
                                n2851 = local read "Mean"() -> (w4630:dbl)
                                n2852 = Greater?(x=w4630, y=11.0) -> (0:w4626:bool)
                                n2853 = Not(x=w4626) -> (.not. x?=w4625:bool)
                                n2854 = And(x=w4626, y=w4627) -> (x .and. y?=w4628:bool)
                                n2855 = And(x=w4625, y=w4627) -> (x .and. y?=w4624:bool)
                                n2856 = case shown="True" w4628 {
                                frame False {
                                }
                                frame True {
                                n2857 = local read "Confocal X 2 (V)"() -> (w4633:dbl)
                                n2858 = local read "Confocal Y 2 (V)"() -> (w4634:dbl)
                                n2859 = property on="AO2" class="Slide (strict)"("Val(Sgnl)"=w4633) -> ()  [unwired: 2 in, 2 out]
                                n2860 = property on="AO1" class="Slide (strict)"("Val(Sgnl)"=w4634) -> ()  [unwired: 2 in, 2 out]
                                }
                                }
                                n2861 = case shown="True" w4624 {
                                frame False {
                                }
                                frame True {
                                n2862 = local read "Confocal Y 1 (V)"() -> (w4632:dbl)
                                n2863 = local read "Confocal X 1 (V)"() -> (w4631:dbl)
                                n2864 = property on="AO1" class="Slide (strict)"("Val(Sgnl)"=w4632) -> ()  [unwired: 2 in, 2 out]
                                n2865 = property on="AO2" class="Slide (strict)"("Val(Sgnl)"=w4631) -> ()  [unwired: 2 in, 2 out]
                                }
                                }
                                }
                                frame #6 {
                                n2866 = Wait (ms)(milliseconds to wait=u32 1500) -> ()  [unwired: 1 out]
                                }
                                frame #7 {
                                n2867 = property on="Rem fb disp offset" class="Bool (strict)"("Val(Sgnl)"=TRUE ("Value (Signaling)")) -> ()  [unwired: 2 in, 2 out]
                                }
                                }
                                }
                                frame True {
                                n2868 = flat-sequence {
                                tunnel: w4637 -> [w4638]
                                frame #0 {
                                n2869 = property on="Trap Delta (MHz)" class="DigNum (strict)"("Val(Sgnl)"=w4638) -> ()  [unwired: 2 in, 2 out]
                                }
                                frame #1 {
                                n2870 = Wait (ms)(milliseconds to wait=u32 500) -> ()  [unwired: 1 out]
                                }
                                frame #2 {
                                n2871 = local read "Shift confocal"() -> (w4644:bool)
                                n2872 = local read "Mean"() -> (w4645:dbl)
                                n2873 = Greater?(x=w4645, y=11.0) -> (0:w4643:bool)
                                n2874 = And(x=w4643, y=w4644) -> (x .and. y?=w4641:bool)
                                n2875 = Not(x=w4643) -> (.not. x?=w4642:bool)
                                n2876 = And(x=w4642, y=w4644) -> (x .and. y?=w4640:bool)
                                n2877 = case shown="True" w4641 {
                                frame False {
                                }
                                frame True {
                                n2878 = local read "Confocal Y 2 (V)"() -> (w4650:dbl)
                                n2879 = local read "Confocal X 2 (V)"() -> (w4649:dbl)
                                n2880 = property on="AO1" class="Slide (strict)"("Val(Sgnl)"=w4650) -> ()  [unwired: 2 in, 2 out]
                                n2881 = property on="AO2" class="Slide (strict)"("Val(Sgnl)"=w4649) -> ()  [unwired: 2 in, 2 out]
                                }
                                }
                                n2882 = case shown="True" w4640 {
                                frame False {
                                }
                                frame True {
